vi "LVClass_Image get image dimensions.vi"(0 "Image in":refnum<class "Image.lvclass">, 11 "error in (no error)":errorcluster) -> (4 "Image out":refnum<class "Image.lvclass">, 6 "Number of pixels":T2, 8 "Number of bits":T1=enum."16", 15 "error out":errorcluster)   [LabVIEW 2020, in "Image.lvclass"]
doc: "Get Image size.\n\n--------------------------------------------------------------------------------\n\n<B>ImageIn </B> : Image object.\n<B>ImageOut </B> : Image object.\n<B>size </B> : Image size (width, height).\n<B>bit_depth </B> : Image bits depth.\n<B>ErrorIn </B> : Error\n<B>ErrorOut </B> : Error\n\n--------------------------------------------------------------------------------"
uses:
  Image.lvclass
  Point2D.ctl
  Data alignment enum.ctl
  Image.lvclass/Image.ctl
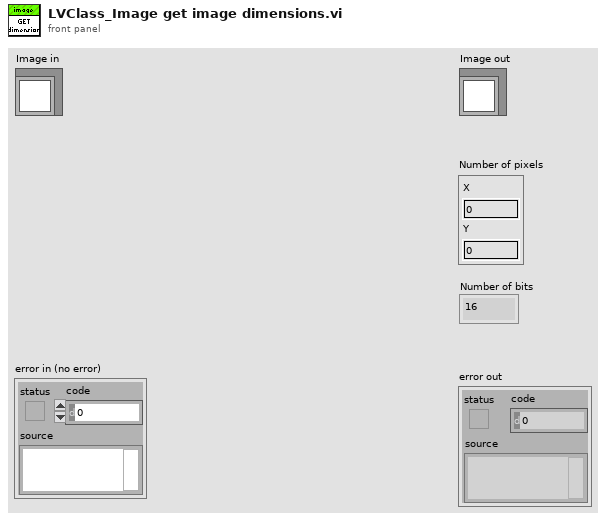
[diagram p1: front panel]
types:
  T1 = typedef "Data alignment enum.ctl" = enum16{"8", "16", "32"}
  T2 = typedef "Point2D.ctl" = cluster{"X":u32, "Y":u32}
  T3 = typedef "ClassID.ctl" = i64
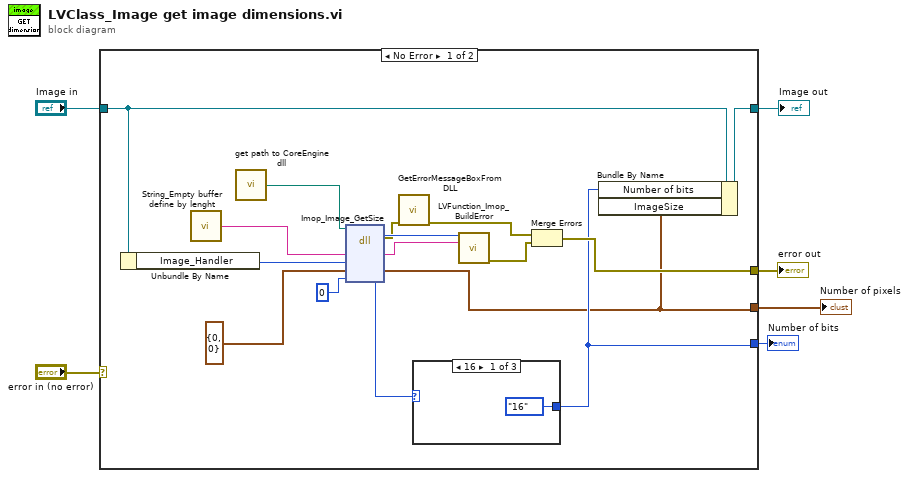
[diagram p0: block diagram]
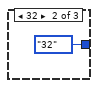
[diagram p2: hidden frame]
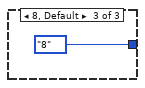
[diagram p3: hidden frame]
diagram:
  n1 = case shown="No Error" "error in (no error)" {
    selector: "error in (no error)" -> [_ w27]
    tunnel: [w12 w27] -> w5
    tunnel: [w8 w26] -> w3
    tunnel: "Image in" -> [w9 w26]
    tunnel: [w10 _] -> w2
    tunnel: [w11 _] -> w1
    frame No Error {
      n2 = Unbundle By Name(w9) -> ("Image_Handler"=w19:T3)
      n3 = call "String_Empty buffer define by lenght.vi"() -> ("Empty buffer"=w22:string)  [unwired: 1 in]
      n4 = call "get path to CoreEngine dll.vi"() -> ("path to wavekit library"=w18:path)  [unwired: 14 in, 1 out]
      n5 = dll-call lib="D:/2_trunk/Soft_haso/ImOpCoreEngine4_LV2011/DLLs/ImopEngine4_vc100.dll" fn="Imop_Image_GetSize"(path in=w18, "message"=w22, "Image compat"=w19, "image_size"=T2 {"X"=0, "Y"=0}, "nb_bits"=u16 0) -> (error out=w16:errorcluster, "return type"=w21:i32, "message"=w20:string, "image_size"=w10:T2, "nb_bits"=w15:u16)  [unwired: 3 in, 1 out]
      n6 = call "GetErrorMessageBoxFromDLL.vi"("error IN"=w16) -> ("error OUT"=w14:errorcluster)  [unwired: 10 in]
      n7 = case shown="16" w15 {
        tunnel: [Data_alignment_enum."16" ("Number of bits") Data_alignment_enum."32" ("Number of bits") Data_alignment_enum."8" ("Number of bits")] -> w11
        frame 16 {
        }
        frame 32 {
        }
        frame 8, Default {
        }
      }
      n8 = call "LVFunction_Imop_BuildError.vi"("code"=w21, "String to Prepend to source (\"\")"=w20) -> ("error out"=w13:errorcluster)  [unwired: 13 in]
      n9 = Merge Errors(w14, w13) -> (w12:errorcluster)
      n10 = Bundle By Name(cluster=w9, "Number of bits"=w11, "ImageSize"=w10) -> (w8:refnum<class "Image.lvclass">)
    }
    frame Error {
    }
  }
  "error out" <- w5
  "Image out" <- w3
  "Number of pixels" <- w2
  "Number of bits" <- w1
